vi "Wifi AP Setting IP.vi"() -> ()   [LabVIEW 2014, in "ESP8266 WiFi Wrapper.lvlib"]
uses:
  <vilib>/Aledyne-TSXperts/Arduino Compatible Compiler for LabVIEW/addons/ESP8266 WiFi Wrapper/ESP8266 WiFi Wrapper.lvlib
  <vilib>/Aledyne-TSXperts/Arduino Compatible Compiler for LabVIEW/Arduino Compatible Compiler for LabVIEW.lvlib
panel:
  out "Error Out":errorcluster
  in  "DNS address":u8[](array[numeric])=[1, 2, 3, 4]
  in  "IP address":u8[](array[numeric])=[192, 168, 0, 42]
  in  "Gateway":u8[](array[numeric])=[192, 168, 0, 1]
  in  "Subnet mask":u8[](array[numeric])=[255, 255, 255, 0]
  in  "Password":string="12345678"
  in  "SSID":string="ESP8266 Wifi Example"
  in  "Listen Port":u8=80
  in  "error in (no error)":errorcluster
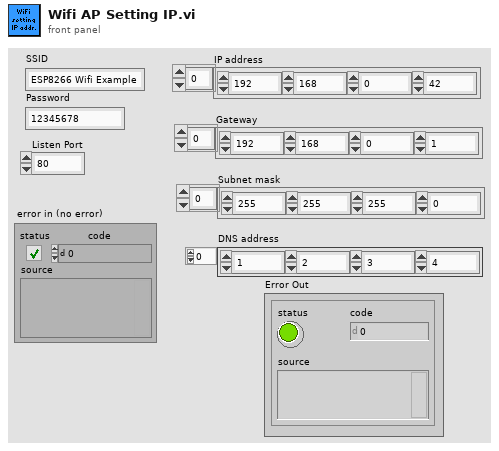
[diagram p1: front panel]
types:
  T1 = enum16{"WIFI_OFF", "WIFI_STA", "WIFI_AP", "WIFI_AP_STA"}
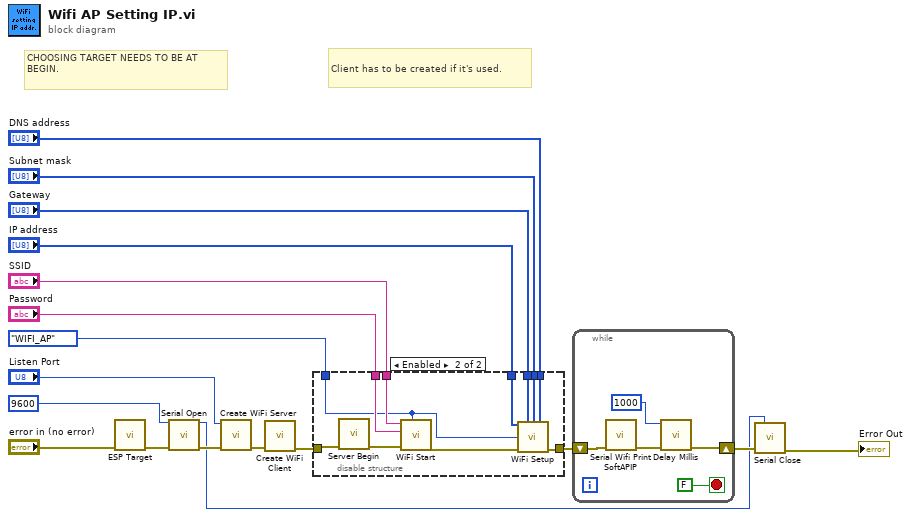
[diagram p0: block diagram]
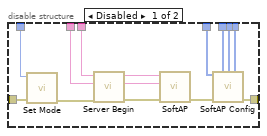
[diagram p2: hidden frame]
diagram:
  # "CHOOSING TARGET NEEDS TO BE AT BEGIN."
  # "Client has to be created if it's used."
  n1 = call <vilib>:"ESP Target.vi"("Error In"="error in (no error)") -> ("Error Out"=w14:errorcluster)  [unwired: 10 in]
  n2 = call <vilib>:"Serial Open.vi"("Speed"=u32 9600, "error in (no error)"=w14) -> ("Instance"=w3:u8, "error out"=w17:errorcluster)  [unwired: 12 in]
  n3 = call <vilib>:"Create WiFi Server.vi"("Error In"=w17, "Listen Port"="Listen Port") -> ("Error Out"=w15:errorcluster)  [unwired: 9 in]
  n4 = call <vilib>:"Create WiFi Client.vi"("Error In"=w15) -> ("Error Out"=w2:errorcluster)  [unwired: 10 in]
  n5 = disable-structure shown="Enabled" {
    disable-tunnel: "DNS address" -> [w30 w35]
    disable-tunnel: "Subnet mask" -> [w29 w34]
    disable-tunnel: "Gateway" -> [w28 w33]
    disable-tunnel: "IP address" -> [w27 w32]
    disable-tunnel: "SSID" -> [w25 w41]
    disable-tunnel: "Password" -> [w24 w40]
    disable-tunnel: [w22 w36] -> w6
    disable-tunnel: w2 -> [w21 w38]
    disable-tunnel: T1."WIFI_AP" ("WiFi Server Mode") -> [w19 w31]
    frame Disabled {
      n6 = call <vilib>:"Set Mode.vi"("Error In"=w21, "WiFi Server Mode"=w19) -> ("Error Out"=w20:errorcluster)  [unwired: 9 in]
      n7 = call <vilib>:"Server Begin.vi"("Error In"=w20) -> ("Error Out"=w23:errorcluster)  [unwired: 10 in]
      n8 = call <vilib>:"SoftAP.vi"("Error In"=w23, "Password"=w24, "SSID"=w25) -> ("Error Out"=w26:errorcluster)  [unwired: 8 in]
      n9 = call <vilib>:"SoftAP Config.vi"("IP address"=w27, "Gateway address"=w28, "Subnet mask"=w29, "DNS address"=w30, "Error In"=w26) -> ("Error Out"=w22:errorcluster)  [unwired: 10 in]
    }
    frame Enabled {
      n10 = call <vilib>:"Server Begin.vi"("Error In"=w38) -> ("Error Out"=w39:errorcluster)  [unwired: 10 in]
      n11 = call <vilib>:"WiFi Start.vi"("WiFi Mode"=w31, "Error In"=w39, "Password"=w40, "SSID"=w41) -> ("Error Out"=w37:errorcluster)  [unwired: 7 in]
      n12 = call <vilib>:"WiFi Setup.vi"("IP address"=w32, "Gateway address"=w33, "Subnet mask"=w34, "DNS address"=w35, "WiFi Mode"=w31, "Error In"=w37) -> ("Error Out"=w36:errorcluster)  [unwired: 9 in]
    }
  }
  n13 = while {
    shift-right: [w44] -> w5
    shift-left: w6 -> [w46]
    stop <- FALSE stop-if-true
    n14 = call <vilib>:"Serial Wifi Print SoftAPIP.vi"("Error In"=w46) -> ("Error Out"=w45:errorcluster)  [unwired: 10 in]
    n15 = call <vilib>:"Delay Millis.vi"("error in (no error)"=w45, "delay"=u32 1000) -> ("error out"=w44:errorcluster)  [unwired: 9 in]
  }
  n16 = call <vilib>:"Serial Close.vi"("Instance"=w3, "error in (no error)"=w5) -> ("error out"=→"Error Out":errorcluster)  [unwired: 13 in]
